vi "waaca_kg.vi"(9 "AC/BD":bool, 11 "Voltage in":dbl) -> (3 "KG output":dbl)   [LabVIEW 2016]
panel:
  # "False = AC\nTrue = BD"
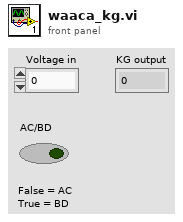
[diagram p1: front panel]
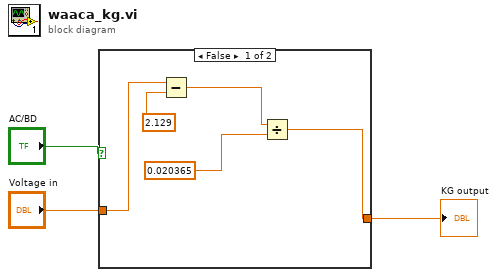
[diagram p0: block diagram]
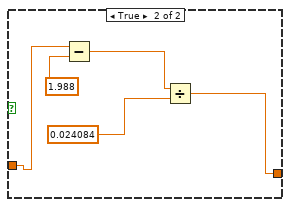
[diagram p2: hidden frame]
diagram:
  n1 = case shown="False" "AC/BD" {
    tunnel: "Voltage in" -> [w6 w10]
    tunnel: [w4 w9] -> w1
    frame False {
      n2 = Subtract(x=w6, y=2.129) -> (x-y=w7:dbl)
      n3 = Divide(x=w7, y=0.020365) -> (x/y=w4:dbl)
    }
    frame True {
      n4 = Subtract(x=w10, y=1.988) -> (x-y=w12:dbl)
      n5 = Divide(x=w12, y=0.024084) -> (x/y=w9:dbl)
    }
  }
  "KG output" <- w1
